vi "_Construct Calibration Table.vi"(7 "Calibration":dbl[][](array[numeric])) -> (1 "Table":string[][](array[string]), 3 "Rows":i32)   [LabVIEW 2012]
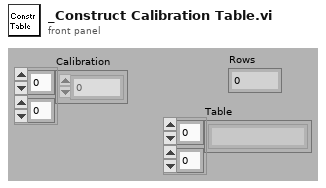
[diagram p1: front panel]
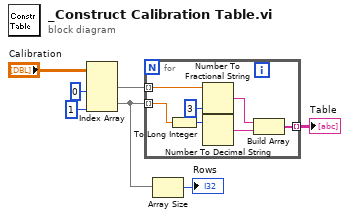
[diagram p0: block diagram]
diagram:
  n1 = Index Array(array="Calibration", index (col) #1=0 ("Index"), index (col) #2=1 ("index (col)")) -> (element #1=w4:dbl[], element #2=w2:dbl[])  [unwired: 2 in]
  n2 = for {
    tunnel: [w11] -> w3 mode=indexing
    tunnel: w4 -> [w9] mode=indexing
    tunnel: w2 -> [w10] mode=indexing
    n3 = To Long Integer(number=w10) -> (32bit integer=w14:i32)
    n4 = Number To Fractional String(number=w9, precision (6)=i16 3) -> (F-format string=w13:string)  [unwired: 2 out]
    n5 = Number To Decimal String(number=w14) -> (decimal integer string=w12:string)  [unwired: 1 out]
    n6 = Build Array(w13, w12) -> (w11:string[])
  }
  "Table" <- w3
  n7 = Array Size(array=w2) -> (size(s)=→"Rows":i32)
